vi "lesson 2_1.vi"() -> ()   [LabVIEW 2013]
panel:
  in  "Numeric":dbl
  out "TRUE":bool
  out "FALSE":bool
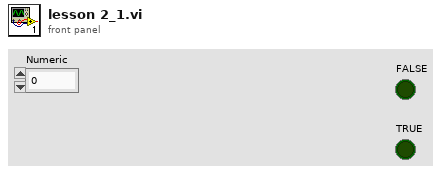
[diagram p1: front panel]
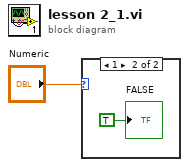
[diagram p0: block diagram]
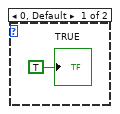
[diagram p2: hidden frame]
diagram:
  n1 = case shown="1" "Numeric" {
    frame 0, Default {
      "TRUE" <- TRUE ("Boolean 3")
    }
    frame 1 {
      "FALSE" <- TRUE ("Boolean 2")
    }
  }
